vi "BIN_PAQ_year_nums_2_filename.vi"(6 "num Stop":u64, 8 "error in":errorcluster, 9 "num Start":u64, 10 "ext":string, 11 "TableName":string) -> (0 "error out":errorcluster, 2 "FileNames":string[](array[string]))   [LabVIEW 2020, in "Sgraph_lib_V1.lvlib" / "DBAL-BIN.lvclass"]
doc: "Binary PAQ file: numeric file identifier to filename\n(array of 1 or two names)"
uses:
  DBAL-BIN.lvclass
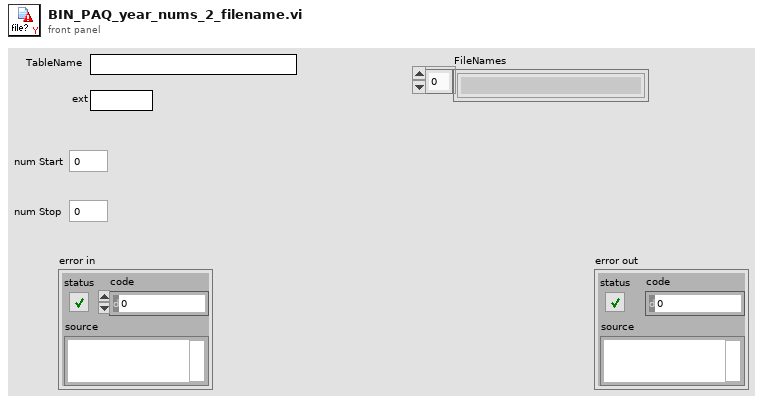
[diagram p1: front panel]
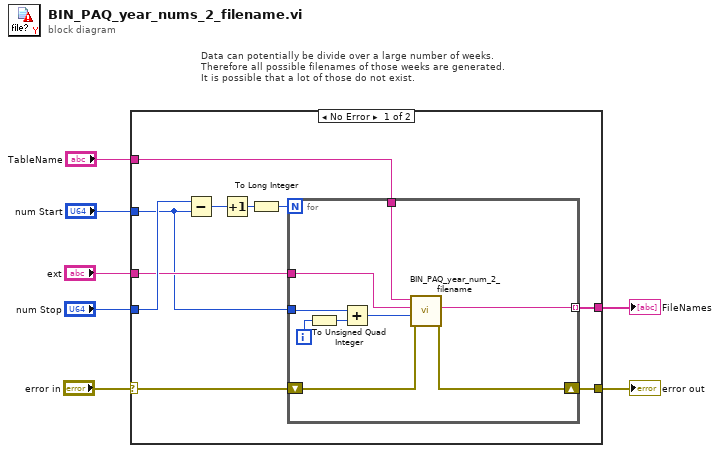
[diagram p0: block diagram]
diagram:
  # "Data can potentially be divide over a large number of weeks.\nTherefore all possible filenames of those weeks are generated.\nIt is possible that a lot of those do not exist."
  n1 = case shown="No Error" "error in" {
    selector: "error in" -> [w11 w27]
    tunnel: "TableName" -> [w13 _]
    tunnel: "ext" -> [w12 _]
    tunnel: "num Start" -> [w8 _]
    tunnel: "num Stop" -> [w14 _]
    tunnel: [w10 _] -> w3
    tunnel: [w9 w27] -> w1
    frame No Error {
      n2 = Subtract(x=w14, y=w8) -> (x-y=w17:u64)
      n3 = Increment(x=w17) -> (x+1=w16:u64)
      n4 = To Long Integer(number=w16) -> (32bit integer=w15:i32)
      n5 = for {
        N: w15 -> [_]
        tunnel: w8 -> [w26]
        tunnel: w13 -> [w22]
        tunnel: w12 -> [w21]
        shift-right: [w19] -> w9
        shift-left: w11 -> [w20]
        tunnel: [w18] -> w10 mode=indexing
        i -> [w25]
        n6 = To Unsigned Quad Integer(1:w25) -> (0:w24:u64)
        n7 = Add(x=w26, y=w24) -> (x+y=w23:u64)
        n8 = call "BIN_PAQ_year_num_2_filename.vi"("error in"=w20, "num"=w23, "ext"=w21, "TableName"=w22) -> ("error out"=w19:errorcluster, "FileName"=w18:string)  [unwired: 6 in]
      }
    }
    frame Error {
    }
  }
  "FileNames" <- w3
  "error out" <- w1
